vi "Electrode Visualization.vi"(8 "error in":errorcluster, 9 "Electrode Type":string="V-", 10 "Electrode Name":string="A") -> (0 "error out":errorcluster, 3 "String A":string)   [LabVIEW 2020, in "Retrieve and Visualize.lvclass"]
uses:
  Retrieve and Visualize.lvclass
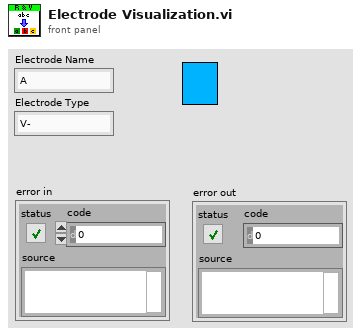
[diagram p1: front panel]
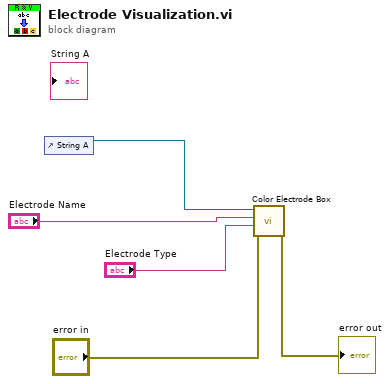
[diagram p0: block diagram]
diagram:
  n1 = control-ref of="String A"() -> (w5:refnum<vi>)
  n2 = call "Color Electrode Box.vi"("error in (no error)"="error in", "Electrode Type"="Electrode Type", "Electrode Name"="Electrode Name", "Reference"=w5) -> ("error out"=→"error out":errorcluster)  [unwired: 7 in]
